vi "2Darray2String_UDP.vi"(2 "NumberOfChannels":i32, 3 "NumberOfSamples":i32, 4 "Waveform Graph":dbl[][](graph)) -> (0 "UDP_StringLength":i32, 1 "UDP_String":string)   [LabVIEW 2015]
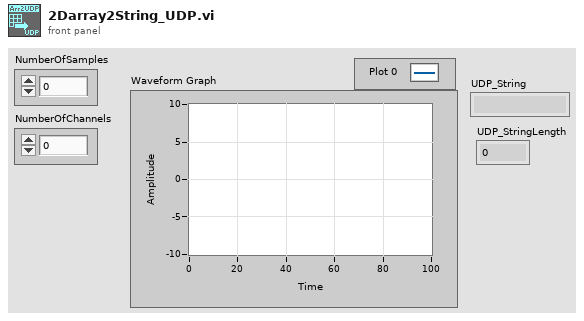
[diagram p1: front panel]
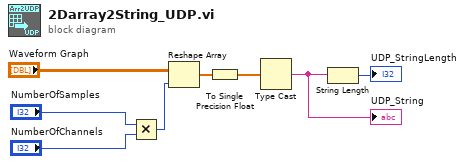
[diagram p0: block diagram]
diagram:
  n1 = Multiply(x="NumberOfSamples", y="NumberOfChannels") -> (x*y=w6:i32)
  n2 = Reshape Array("Waveform Graph", w6) -> (w5:dbl[])
  n3 = To Single Precision Float(number=w5) -> (single precision float=w4:sgl[])
  n4 = Type Cast(x=w4) -> (*(type *) &x=w2:string)  [unwired: 1 in]
  "UDP_String" <- w2
  n5 = String Length(string=w2) -> (length=→"UDP_StringLength":i32)
